vi "StopAOVoltage.vi"   [LabVIEW 2012]
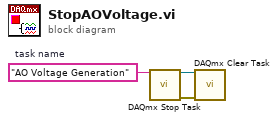
[diagram p0: block diagram]
diagram:
  w1 = "AO Voltage Generation"  # task name
  n1 = call <vilib>:"DAQmx Stop Task.vi"("task/channels in"=w1) -> ("task out"=w2:refnum<k21>, "error out"=w3:errorcluster)  [unwired: 13 in]
  n2 = call <vilib>:"DAQmx Clear Task.vi"("task in"=w2, "error in"=w3) -> ()  [unwired: 13 in, 1 out]
